vi "[FPGA] Single-Phase PLL with Frequency and Amplitude no LPF (FXP).vi"(0 "input":fxp<+/-,16,9>, 1 "reset":bool, 5 "Ts":fxp<+,20,-12>=2.998858690261841e-06, 7 "2*Mu1":fxp<+,10,10>=200.0, 9 "2*Mu2":fxp<+/-,16,16>=6000.0, 11 "u3":fxp<+/-,16,1>=0.010009765625, 12 "fc":fxp<+/-,16,8>=60.0) -> (3 "frequency (Hz)":fxp<+,20,10> format="%#.6g", 4 "phase (pi)":fxp<+/-,16,1> format="%#.6g", 6 "sin(phase)":fxp<+/-,16,2> format="%#.6g", 8 "Vgrid_PLL":fxp<+/-,24,9>, 10 "cos(phase)":fxp<+/-,16,2> format="%#.6g", 15 "amplitude":fxp<+/-,24,9> format="%#.6g")   [LabVIEW 2015]
uses:
  <vilib>/rvi/FXPMathLib/FxpSinAndCos/subVIs/nifxpmath_SinAndCos_SimConfig.ctl
  <vilib>/rvi/FXPMathLib/FxpSinAndCos/simVIs/DllFxpSinAndCosTemp_sub.vi
  <vilib>/rvi/FXPMathLib/FxpSinAndCos/XNode/nifxpmath_SinAndCos.xnode
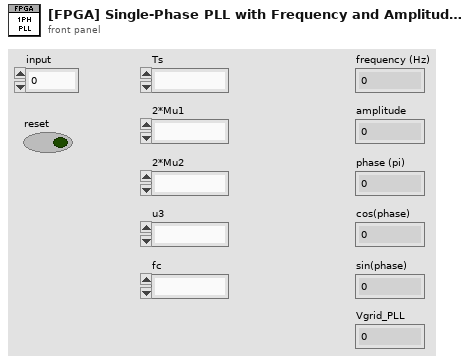
[diagram p1: front panel]
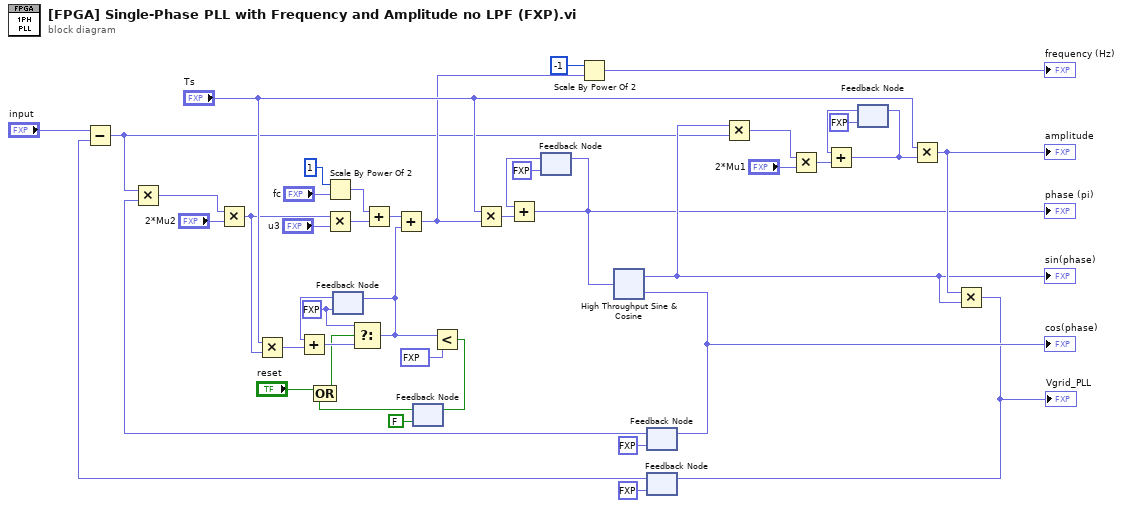
[diagram p0: block diagram]
diagram:
  w10 = fxp<+/-,32,10> 0.0
  n1 = Scale By Power Of 2(n=1, x="fc") -> (x*2^n=w28:fxp<+/-,16,8>)
  n2 = feedback #1(w10) -> (w34:fxp<+/-,32,10>)
  n3 = feedback #2(FALSE) -> (w6:bool)
  n4 = Compound Arithmetic op=OR("reset", w6) -> (w5:bool)
  n5 = feedback #3(fxp<+/-,32,1> 0.0) -> (w17:fxp<+/-,32,1>)
  n6 = feedback #4(fxp<+/-,32,2> 0.0 ("cos(x)")) -> (w37:fxp<+/-,32,2>)
  n7 = feedback #5(fxp<+/-,24,9> 0.0) -> (w38:fxp<+/-,24,9>)
  n8 = Subtract(x="input", y=w38) -> (x-y=w19:fxp<+/-,25,10>)
  n9 = Multiply(x=w19, y=w37) -> (x*y=w20:fxp<+/-,32,11>)
  n10 = Multiply(x=w20, y="2*Mu2") -> (x*y=w21:fxp<+/-,32,26>)
  n11 = Multiply(x="Ts", y=w21) -> (x*y=w18:fxp<+/-,32,4>)
  n12 = Add(x=w34, y=w18) -> (x+y=w11:fxp<+/-,32,10>)
  n13 = Multiply(x=w21, y="u3") -> (x*y=w22:fxp<+/-,48,27>)
  n14 = Select(t=w10, s=w5, f=w11) -> (s? t:f=w9:fxp<+/-,32,10>)
  n15 = feedback-in #1(w9) -> ()
  n16 = Add(x=w28, y=w22) -> (x+y=w24:fxp<+/-,48,27>)
  n17 = Add(x=w24, y=w9) -> (x+y=w23:fxp<+,32,10>)
  n18 = Less?(x=w9, y=fxp<+/-,32,10> -120.0) -> (x < y?=w3:bool)
  n19 = feedback-in #2(w3) -> ()
  n20 = Multiply(x="Ts", y=w23) -> (x*y=w32:fxp<+,32,-6>)
  n21 = Add(x=w17, y=w32) -> (x+y=w16:fxp<+/-,32,1>)
  "phase (pi)" <- w16
  n22 = feedback-in #3(w16) -> ()
  n23 = Scale By Power Of 2(n=-1, x=w23) -> (x*2^n=→"frequency (Hz)":fxp<+,32,10>)
  n24 = xnode "High Throughput Sine & Cosine"("x (pi)"=w16) -> ("sin(x)"=w31:fxp<+/-,32,2>, "cos(x)"=w30:fxp<+/-,32,2>)
  "cos(phase)" <- w30
  "sin(phase)" <- w31
  n25 = feedback-in #4(w30) -> ()
  n26 = Multiply(x=w31, y=w19) -> (x*y=w42:fxp<+/-,16,10>)
  n27 = Multiply(x=w42, y="2*Mu1") -> (x*y=w26:fxp<+/-,26,20>)
  n28 = feedback #6(fxp<+/-,36,28> 0.0) -> (w41:fxp<+/-,36,28>)
  n29 = Add(x=w41, y=w26) -> (x+y=w40:fxp<+/-,36,28>)
  n30 = feedback-in #6(w40) -> ()
  n31 = Multiply(x="Ts", y=w40) -> (x*y=w39:fxp<+/-,24,9>)
  "amplitude" <- w39
  n32 = Multiply(x=w39, y=w31) -> (x*y=w2:fxp<+/-,24,9>)
  "Vgrid_PLL" <- w2
  n33 = feedback-in #5(w2) -> ()
